vi "Set Shared Variable Refnum.vi"(8 "error in (no error)":errorcluster, 10 "shared variable refnum":refnum<k21>, 11 "abs_SharedVar_Bool in":refnum<class "conc_SharedVar_U64.lvclass">) -> (0 "error out":errorcluster, 3 "abs_SharedVar_Bool out":refnum<class "conc_SharedVar_U64.lvclass">)   [LabVIEW 2021, in "conc_SharedVar_U64.lvclass"]
doc: "LVabs_Shared Variable 1.0.0.2\nTim - TSA\nCopyright (c) 2024, TSA"
uses:
  conc_SharedVar_U64.lvclass
  conc_SharedVar_U64.lvclass/conc_SharedVar_U64.ctl
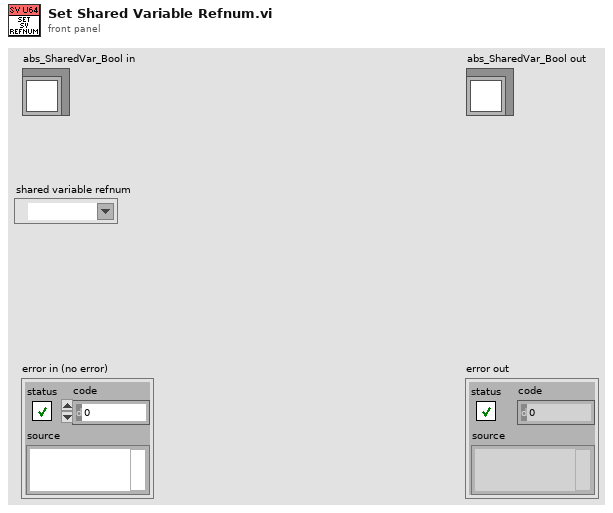
[diagram p1: front panel]
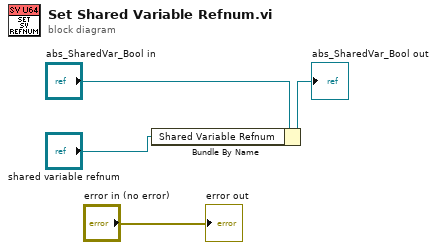
[diagram p0: block diagram]
diagram:
  n1 = Bundle By Name(cluster="abs_SharedVar_Bool in", "Shared Variable Refnum"="shared variable refnum") -> (→"abs_SharedVar_Bool out":refnum<class "conc_SharedVar_U64.lvclass">)
  "error out" <- "error in (no error)"
